vi "Configure Filter.vi"(6 "Filter Time (s) (2)":dbl=2.0 min=0.0125 max=100.0 step=1.0, 7 "Channel (0: Channel A)":u16(ring) items=["Channel A", "Channel B"], 8 "error in (no error)":errorcluster, 9 "Filter Band %FS (0.02)":dbl=0.02 min=0.0 max=100.0 step=0.01, 10 "Enable Filter (Off)":bool, 11 "BH Druck PACE Series in":refnum<class "BH Druck PACE Series.lvclass">) -> (0 "error out":errorcluster, 3 "BH Druck PACE Series out":refnum<class "BH Druck PACE Series.lvclass">)   [LabVIEW 2022 SP3, in "BH Druck PACE Series.lvclass"]
uses:
  BH Druck PACE Series.lvclass
  BH Druck PACE Series.lvclass/BH Druck PACE Series.ctl
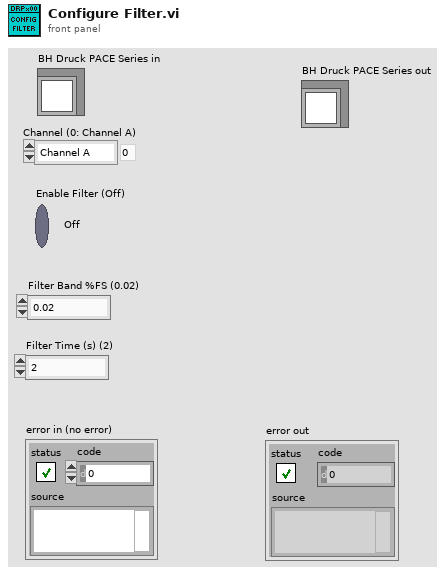
[diagram p1: front panel]
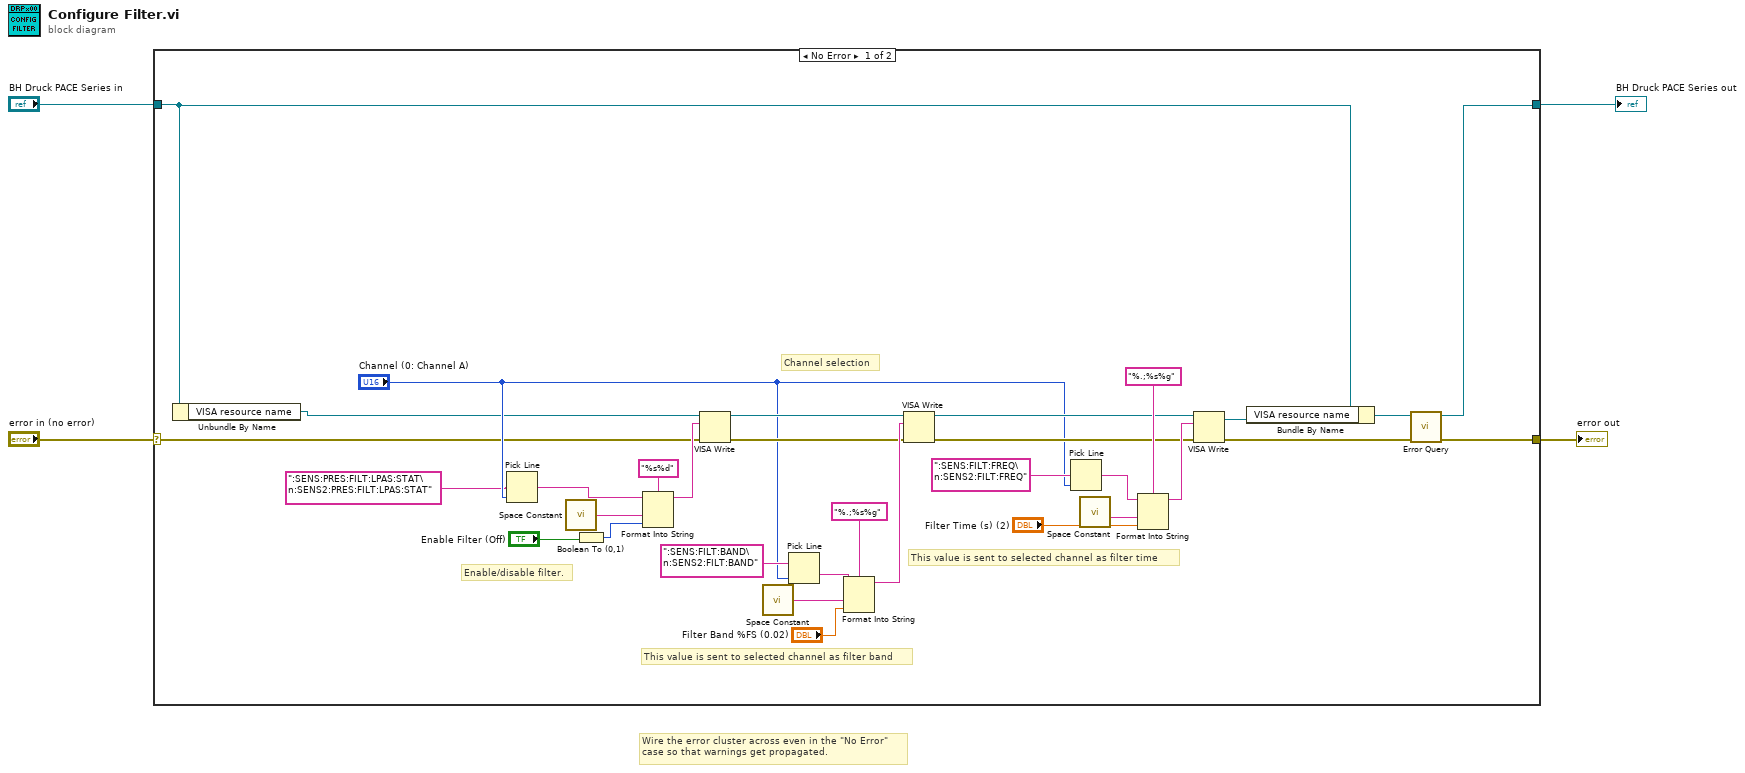
[diagram p0: block diagram]
diagram:
  # "Wire the error cluster across even in the \"No Error\"\ncase so that warnings get propagated."
  n1 = case shown="No Error" "error in (no error)" {
    selector: "error in (no error)" -> [w13 w38]
    tunnel: [w6 w38] -> w3
    tunnel: [w5 w37] -> w1
    tunnel: "BH Druck PACE Series in" -> [w9 w37]
    frame No Error {
      # "This value is sent to selected channel as filter time"
      # "This value is sent to selected channel as filter band"
      # "Enable/disable filter."
      # "Channel selection"
      n2 = Unbundle By Name(w9) -> ("VISA resource name"=w12:refnum<visa-resource-name>)
      n3 = Pick Line(multi-line string=":SENS:PRES:FILT:LPAS:STAT\n:SENS2:PRES:FILT:LPAS:STAT", line index="Channel (0: Channel A)") -> (output string=w34:string)  [unwired: 1 in]
      n4 = call <vilib>:"Space Constant.vi"() -> ("String"=w32:string)
      n5 = Boolean To (0,1)(Boolean="Enable Filter (Off)") -> (0, 1=w33:i16)
      n6 = Format Into String(format string="%s%d", initial string=w34, w32, w33) -> (resulting string=w35:string)  [unwired: 1 in, 1 out]
      n7 = VISA Write(VISA resource name=w12, write buffer=w35, error in (no error)=w13) -> (VISA resource name out=w24:refnum<visa-resource-name>, error out=w23:errorcluster)  [unwired: 1 out]
      n8 = call <vilib>:"Space Constant.vi"() -> ("String"=w27:string)
      n9 = Pick Line(multi-line string=":SENS:FILT:BAND\n:SENS2:FILT:BAND", line index="Channel (0: Channel A)") -> (output string=w28:string)  [unwired: 1 in]
      n10 = Format Into String(format string="%.;%s%g", initial string=w28, w27, "Filter Band %FS (0.02)") -> (resulting string=w29:string)  [unwired: 1 in, 1 out]
      n11 = VISA Write(VISA resource name=w24, write buffer=w29, error in (no error)=w23) -> (VISA resource name out=w16:refnum<visa-resource-name>, error out=w15:errorcluster)  [unwired: 1 out]
      n12 = Pick Line(multi-line string=":SENS:FILT:FREQ\n:SENS2:FILT:FREQ", line index="Channel (0: Channel A)") -> (output string=w22:string)  [unwired: 1 in]
      n13 = call <vilib>:"Space Constant.vi"() -> ("String"=w18:string)
      n14 = Format Into String(format string="%.;%s%g", initial string=w22, w18, "Filter Time (s) (2)") -> (resulting string=w20:string)  [unwired: 1 in, 1 out]
      n15 = VISA Write(VISA resource name=w16, write buffer=w20, error in (no error)=w15) -> (VISA resource name out=w8:refnum<visa-resource-name>, error out=w10:errorcluster)  [unwired: 1 out]
      n16 = Bundle By Name(cluster=w9, "VISA resource name"=w8) -> (w7:refnum<class "BH Druck PACE Series.lvclass">)
      n17 = call-dynamic "Error Query.vi"("error in (no error)"=w10, "BH Druck PACE Series in"=w7) -> ("error out"=w6:errorcluster, "BH Druck PACE Series out"=w5:refnum<class "BH Druck PACE Series.lvclass">)  [unwired: 8 in]
    }
    frame Error {
    }
  }
  "error out" <- w3
  "BH Druck PACE Series out" <- w1
